vi "Report Gen Sections.vi"(8 "error in (no error)":errorcluster, 11 "report":T1) -> (0 "error out":errorcluster, 3 "report out":T1)   [LabVIEW 2020, in "WebServiceImporter.lvlib" / "Error Handling.lvlib"]
uses:
  <vilib>/Platform/WebService/Error Handling/Error Handling.lvlib
  <resource>/importtools/NISH Report/Generate Report Object Reference.ctl
  <vilib>/Platform/WebService/Error Handling/Error/Operation.ctl
  <vilib>/Platform/WebService/Global/Const Strings.vi
  <vilib>/Platform/WebService/WebServiceImporter.lvlib
  <resource>/importtools/NISH Report/NISH Report.lvlib
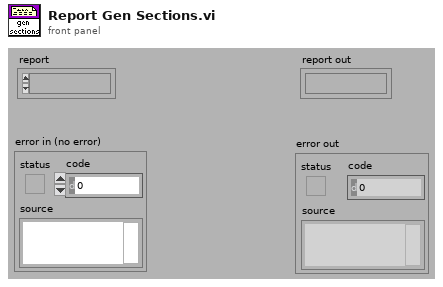
[diagram p1: front panel]
types:
  T1 = typedef "NISH Report.lvlib/Generate Report Object Reference.ctl" = refnum<k1>
  T2 = typedef "WebServiceImporter.lvlib/Error Handling.lvlib/Operation.ctl" = enum16{"Get", "Add", "Clear"}
  T3 = typedef "WebServiceImporter.lvlib/Error Handling.lvlib/Error Info.ctl" = cluster{"Specifics":string, "Error Number":T4, "Call Chain":string, "Context":T5}
  T4 = typedef "WebServiceImporter.lvlib/Error Handling.lvlib/Error Number.ctl" = u16
  T5 = typedef "WebServiceImporter.lvlib/Error Handling.lvlib/Context.ctl" = cluster{"name":T6, "value":string}[]
  T6 = typedef "WebServiceImporter.lvlib/Error Handling.lvlib/Context Name.ctl" = u16
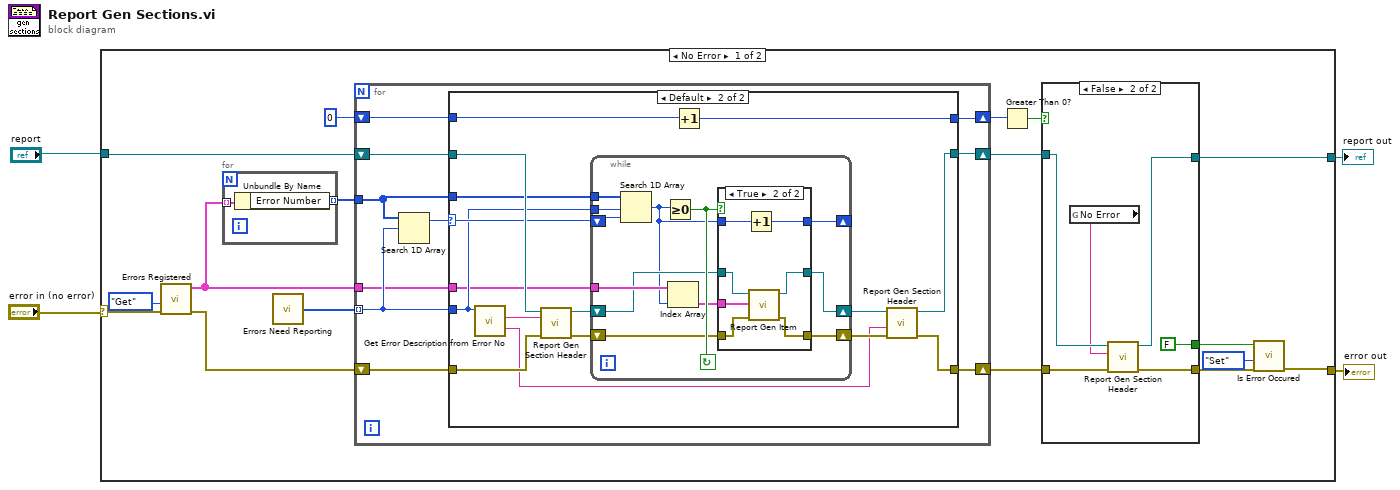
[diagram p0: block diagram]
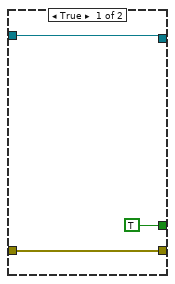
[diagram p2: hidden frame]
diagram:
  n1 = case shown="No Error" "error in (no error)" {
    selector: "error in (no error)" -> [w21 w84]
    tunnel: "report" -> [w18 w85]
    tunnel: [w6 w84] -> w2
    tunnel: [w10 w85] -> w1
    frame No Error {
      n2 = call <vilib>:"Errors Registered.vi"("error in (no error)"=w21, "Operation"=Operation."Get") -> ("error out"=w16:errorcluster, "Array (out)"=w15:T3[])  [unwired: 8 in]
      n3 = for {
        tunnel: w15 -> [w32] mode=indexing
        tunnel: [w31] -> w17 mode=indexing
        n4 = Unbundle By Name(w32) -> ("Error Number"=w31:T4)
      }
      n5 = call <vilib>:"Errors Need Reporting.vi"() -> ("Errors Need Reporting"=w9:T4[])
      n6 = for {
        shift-right: [w33] -> w14
        shift-left: 0 -> [w34]
        tunnel: w9 -> [w39] mode=indexing
        tunnel: w17 -> [w38]
        shift-right: [w36] -> w11
        shift-left: w16 -> [w41]
        tunnel: w15 -> [w37]
        shift-right: [w35] -> w12
        shift-left: w18 -> [w40]
        n7 = Search 1D Array(1D array=w38, element=w39) -> (index of element=w42:i32)  [unwired: 1 in]
        n8 = case shown="Default" w42 {
          selector: w42 -> [_ w57]
          tunnel: w41 -> [w45 w60]
          tunnel: w40 -> [w44 w59]
          tunnel: w39 -> [_ w56]
          tunnel: w38 -> [_ w58]
          tunnel: w37 -> [_ w55]
          tunnel: [w45 w47] -> w36
          tunnel: [w44 w49] -> w35
          tunnel: w34 -> [w43 w52]
          tunnel: [w43 w51] -> w33
          frame -1 {
          }
          frame Default {
            n9 = call <vilib>:"Get Error Description from Error No.vi"("Error Number"=w56) -> ("Error Description"=w46:string, "Error Title"=w61:string)  [unwired: 8 in, 1 out]
            n10 = call <vilib>:"Report Gen Section Header.vi"("error in (no error)"=w60, "Section Title"=w61, "report"=w59) -> ("error out"=w54:errorcluster, "report out"=w53:T1)  [unwired: 7 in]
            n11 = while {
              tunnel: w58 -> [w73]
              shift-right: [w65] -> _
              shift-left: w57 -> [w72]
              tunnel: w56 -> [w71]
              tunnel: w55 -> [w70]
              shift-right: [w63] -> w48
              shift-left: w54 -> [w64]
              shift-right: [w62] -> w50
              shift-left: w53 -> [w67]
              stop <- w69 continue-if-true
              n12 = Search 1D Array(1D array=w73, element=w71, start index (0)=w72) -> (index of element=w66:i32)
              n13 = Greater Or Equal To 0?(x=w66) -> (x >= 0?=w69:bool)
              n14 = Index Array(array=w70, index=w66) -> (element=w68:T3)
              n15 = case shown="True" w69 {
                tunnel: w68 -> [_ w80]
                tunnel: w67 -> [w74 w79]
                tunnel: w66 -> [w76 w83]
                tunnel: [w76 w82] -> w65
                tunnel: w64 -> [w75 w81]
                tunnel: [w74 w78] -> w62
                tunnel: [w75 w77] -> w63
                frame False {
                }
                frame True {
                  n16 = Increment(x=w83) -> (x+1=w82:i32)
                  n17 = call <vilib>:"Report Gen Item.vi"("error in (no error)"=w81, "Error Info"=w80, "report"=w79) -> ("error out"=w77:errorcluster, "report out"=w78:T1)  [unwired: 7 in]
                }
              }
            }
            n18 = Increment(x=w52) -> (x+1=w51:i32)
            n19 = call <vilib>:"Report Gen Section Header.vi"("error in (no error)"=w48, "Section Text"=w46, "report"=w50) -> ("error out"=w47:errorcluster, "report out"=w49:T1)  [unwired: 7 in]
          }
        }
      }
      n20 = Greater Than 0?(x=w14) -> (x > 0?=w13:bool)
      n21 = case shown="False" w13 {
        tunnel: w12 -> [w24 w29]
        tunnel: w11 -> [w23 w30]
        tunnel: [w24 w28] -> w10
        tunnel: [w23 w27] -> w7
        tunnel: [TRUE ("Error Occured?") FALSE ("Error Occured?")] -> w5
        frame True {
        }
        frame False {
          n22 = global read "Const Strings.vi" "No Error"() -> (w26:string)
          n23 = call <vilib>:"Report Gen Section Header.vi"("error in (no error)"=w30, "Section Title"=w26, "report"=w29) -> ("error out"=w27:errorcluster, "report out"=w28:T1)  [unwired: 7 in]
        }
      }
      n24 = call <vilib>:"Is Error Occured.vi"("error in (no error)"=w7, "Enum"=enum16{"Get", "Set"}."Set", "Error Occured?"=w5) -> ("error out"=w6:errorcluster)  [unwired: 7 in, 1 out]
    }
    frame Error {
    }
  }
  "report out" <- w1
  "error out" <- w2
